vi "niFPGA Handshake Pipe Input Control.vi"(7 "reset":bool, 10 "input valid":bool, 11 "ready for input":bool) -> (0 "input buffer enable":bool, 1 "Input Mux Sel":bool, 2 "output valid":bool)   [LabVIEW 2017]
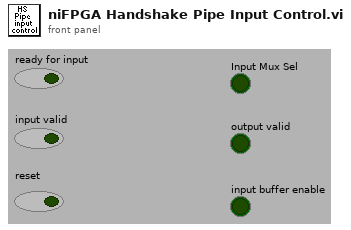
[diagram p1: front panel]
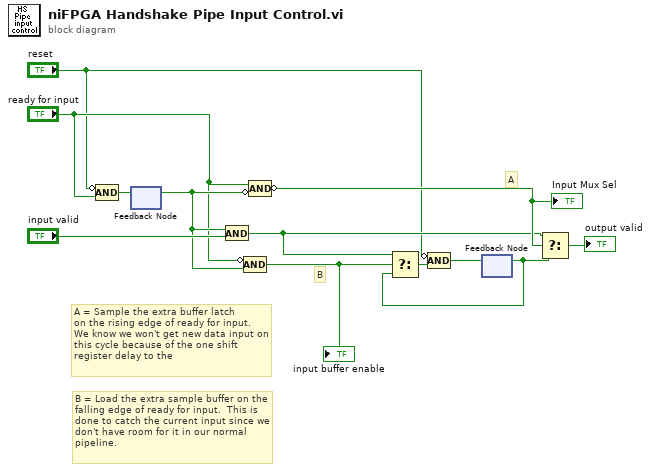
[diagram p0: block diagram]
diagram:
  # "B = Load the extra sample buffer on the falling edge of ready for input.  This is done to catch the current input since we don't have room for it in our normal pipeline."
  # "A = Sample the extra buffer latch\non the rising edge of ready for input.\nWe know we won't get new data input on this cycle because of the one shift register delay to the"
  # "B"
  # "A"
  n1 = Compound Arithmetic op=AND(invert "reset", "ready for input") -> (w5:bool)
  n2 = feedback-in #1(w5) -> ()
  n3 = feedback #1() -> (w7:bool)  [unwired: 1 in]
  n4 = And(x=w7, y="input valid") -> (x .and. y?=w11:bool)
  n5 = Compound Arithmetic op=AND(invert "ready for input", w7) -> (w10:bool)
  "input buffer enable" <- w10
  n6 = Compound Arithmetic op=AND("ready for input", invert w7) -> (invert w12:bool)
  "Input Mux Sel" <- w12
  n7 = feedback #2() -> (w6:bool)  [unwired: 1 in]
  n8 = Select(t=w11, s=w10, f=w6) -> (s? t:f=w3:bool)
  n9 = Compound Arithmetic op=AND(invert "reset", w3) -> (w1:bool)
  n10 = feedback-in #2(w1) -> ()
  n11 = Select(t=w11, s=w12, f=w6) -> (s? t:f=→"output valid":bool)
